vi "General Error Handler.vi"(0 "[error code] (0)":i32 caption="[Fehlercode] (0)" format="%0.0f", 1 "[user-defined codes]":i32[](array[numeric]) caption="[Benutzerspezif. Codes]", 2 "[user-defined descriptions]":string[](array[string]) caption="[Benutzerspezif. Beschreibungen]", 5 "[error source] (\" \")":string caption="[Fehlerquelle] (\" \")", 9 "type of dialog (OK msg:1)":T1=1 caption="Dialog-Typ (OK msg:1)" items=["Kein Dialog", "OK-Nachricht", "Dialog zum Fortsetzen oder Anhalten", "OK Nachricht + Warnungen", "Weiter/Stop + Warnung"], 11 "error in (no error)":errorcluster caption="Fehler (Eingang, kein Fehler)", 12 "[exception action] (none:0)":i32(ring) caption="[Ausnahmeaktion] (none:0)" items=["Keine Ausnahme", "Bei Übereinstimmung Fehler ignorieren", "bei Übereinstimmung Fehler ausgeben"], 13 "[exception code]":i32 caption="[Ausnahmecode]" format="%0.0f", 14 "[exception source]":string caption="[Ausnahmequelle]") -> (4 "error?":bool caption="Fehler?", 6 "code out":i32 caption="Code (Ausgabe)" format="%0.0f", 8 "source out":string caption="Quelle (Ausgang)", 10 "message":string=" INSTRUKTIONEN:\r\rAllgemeine Nutzung:  Bei der Benutzung von SubVIs, die die Fehler(Eingang)-/Fehler(Ausgang)- (oder Fehler-I/O-) Struktur verwenden, plazieren Sie diesen Handler dort, wo Sie den Benutzer auf aufgetretene Fehler hinweisen wollen, typischerweise geschieht dies am Ende eines I/O-Datenpfades als letzte Aktion des Programms.  Wenn der Fehlerstatus einen Fehler angibt, erzeugt der Handler eine Nachricht, die den Fehler und dessen Ursprung beschreibt.  Ist Dialogtyp = 1 (Voreinstellung), wird die Fehlermeldung angezeigt und der Benutzer kann diese lediglich bestätigen.  Ist Dialogtyp = 2, kann der Benutzer die Meldung bestätigen oder die Programm-Ausführung abbrechen; der Abbruch eines Programms mit aktiver I/O wird jedoch nicht empfohlen.  Ist der Dialogtyp = 0, wird keine Meldung angezeigt; dieser Modus wird verwendet, um Fehler programmatisch zu behandeln, aus diesem Grunde sind auch die Fehlerausgangs-Cluster mit individuellen Terminals verbunden.  \r\rAndere Nutzungsmöglichkeit:\n\r\nLokales Testen.  Um einen Fehlercode eines SubVI oder einer Funktion zu testen, die keine Fehler-I/O-Struktur beinhalten, kann deren Fehlercode und ein Quellen-String mit den lokalen Fehlercode- und Quellenstring-Eingängen verbunden werden.  Wenn der Fehlerstatus keinen Fehler anzeigt und der Fehlercode ungleich 0 ist, werden der lokale Code und der String des Fehlereingangs-Wertes ersetzt und Fehler? wird auf TRUE (FEHLER) gesetzt." caption="Meldung", 15 "error out":errorcluster caption="Fehler (Ausgang)")   [LabVIEW 2009]
doc: "Zeigt an, ob ein Fehler aufgetreten ist. Wenn ja, gibt dieses VI eine Fehlermeldung zurück und zeigt (optional) ein Dialogfenster an."
uses:
  DialogType.ctl
  DialogTypeEnum.ctl
panel:
  # "Reinitialisieren auf Standardwerte, um Anweisungen anzuzeigen."
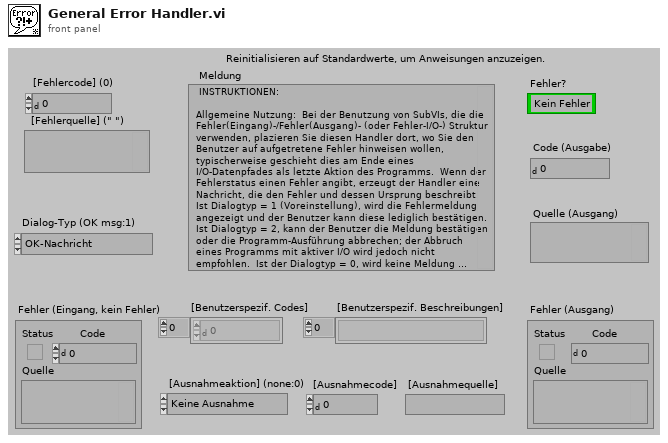
[diagram p1: front panel]
types:
  T1 = typedef "DialogType.ctl" = u16
  T2 = typedef "DialogTypeEnum.ctl" = enum16{"no dialog", "OK message", "continue or stop message", "auto error handling dialog", "OK message + warnings", "continue/stop + warnings"}
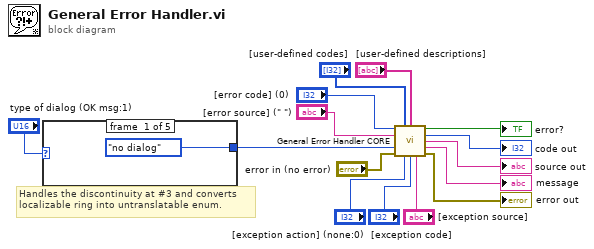
[diagram p0: block diagram]
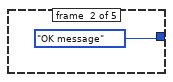
[diagram p2: hidden frame]
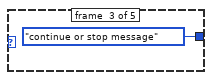
[diagram p3: hidden frame]
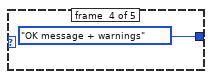
[diagram p4: hidden frame]
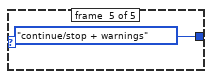
[diagram p5: hidden frame]
diagram:
  # "Handles the discontinuity at #3 and converts\nlocalizable ring into untranslatable enum."
  n1 = case shown="1" "type of dialog (OK msg:1)" {
    tunnel: [DialogTypeEnum."no dialog" ("type of dialog (OK msg:1)") DialogTypeEnum."OK message" ("type of dialog (OK msg:1)") DialogTypeEnum."continue or stop message" ("type of dialog (OK msg:1)") DialogTypeEnum."OK message + warnings" ("type of dialog (OK msg:1)") DialogTypeEnum."continue/stop + warnings" ("type of dialog (OK msg:1)")] -> w1
    frame #0 {
    }
    frame #1 {
    }
    frame #2 {
    }
    frame #3 {
    }
    frame #4 {
    }
  }
  n2 = call "General Error Handler CORE.vi"("[error code] (0)"="[error code] (0)", "[user-defined codes]"="[user-defined codes]", "[user-defined descriptions]"="[user-defined descriptions]", "[error source] (\" \")"="[error source] (\" \")", "type of dialog (OK msg:1)"=w1, "error in (no error)"="error in (no error)", "[exception action] (none:0)"="[exception action] (none:0)", "[exception code]"="[exception code]", "[exception source]"="[exception source]") -> ("error?"=→"error?":bool, "code out"=→"code out":i32, "source out"=→"source out":string, "message"=→"message":string, "error out"=→"error out":errorcluster)  [unwired: 1 in, 1 out]
